vi "GUI_laptop v11c.vi"() -> ()   [LabVIEW 2019]
uses:
  <vilib>/Math Plots/3D Math Plots/3D Scatter/3D Scatter XCtrl/3D Scatter.xctl
  <vilib>/Platform/TimedLoop/XDataNode/timing_clust.ctl
  <vilib>/Platform/TimedLoop/XDataNode/nitl_modes.ctl
  <vilib>/Platform/TimedLoop/XDataNode/wakeup.ctl
  <vilib>/Analysis/_algsub.llb/Real Vector Norm.vi
  <vilib>/Instr/_visa.llb/VISA Configure Serial Port (Instr).vi
  <vilib>/Utility/file.llb/Write Delimited Spreadsheet (DBL).vi
  <vilib>/Math Plots/3D Math Plots/3D Scatter/3D Scatter Datatype/Public/Plot Helper (Vector).vi
  <vilib>/platform/TimedLoop/XDataNode/XDataNode.xnode
  <vilib>/Platform/TimedLoop/XDataNode/XDNodeRunTimeDep.lvlib
  <vilib>/Analysis/NI_AALPro.lvlib
  <vilib>/Math Plots/3D Math Plots/3D Scatter/3D Scatter Datatype/3D Scatter Datatype.lvclass
panel:
  in  "Motion Scale 4":dbl=2.0
  out "spreadsheet string":string
  out "1-D Array of Real 2":dbl[](array[numeric])
  out "1-D Array of Real":dbl[](array[numeric])
  in  "Save Path 2":path=path "C:/Users/jimmy/Documents/GitHub/Arduino-LabVIEW/zhantao/read_data_delt.csv"
  out "Numeric":i32
  out "send values":dbl[](array[numeric])
  out "Robot Feedback (xyz)":dbl[](array[numeric])
  in  "UDP Send":bool
  in  "UDP Recv":bool
  in  "L5 bound":dbl=1000.0
  in  "L4 bound (deg)":dbl=1000.0
  in  "L3 bound (mm)":dbl=1000.0
  in  "L2 bound (deg)":dbl=1000.0
  in  "L1 bound (deg)":dbl=1000.0
  in  "Joystick Type":dbl(ring) items=["Rigid Joystick", "Free Joystick"]
  out "Finished Late? [i-1]":bool
  in  "Epsilon":dbl=0.2
  out "3D Scatter":refnum<class "3D Plot Datatype.lvclass">[](xcontrol)
  out "Random Point":dbl[](array[numeric])
  out "Virtual Cursor":dbl[](array[numeric])
  out "Iteration Duration":i64
  in  "Num of Points":i32=10
  in  "z bound":dbl=2.0
  in  "y bound":dbl=5.0
  in  "x bound":dbl=5.0
  in  "Stop":bool
  in  "Round Decimals":dbl=2.0 format="%#_15g"
  in  "Save  Data":bool
  in  "Save Path":path=path "C:/Users/jimmy/Documents/GitHub/Arduino-LabVIEW/zhantao/read_data_abs.csv"
  in  "x speed":dbl=0.5
  in  "z speed":dbl=0.5
  in  "y speed":dbl=0.5
  out "error out":errorcluster
  in  "baud rate":u32=115200
  in  "VISA resource name":refnum<visa-resource-name>
  # "TODO: fix the bounds; currently bounds are arbitrary"
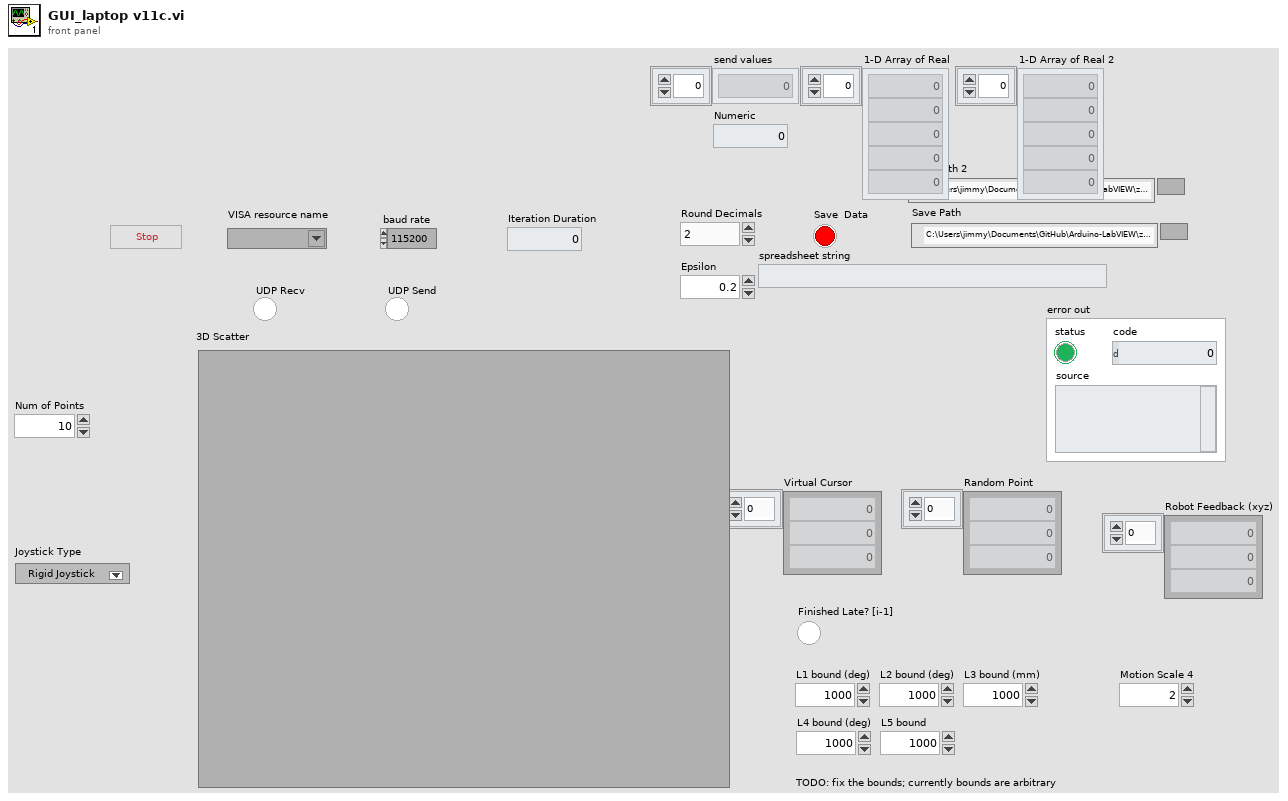
[diagram p1: front panel]
types:
  T1 = typedef "XDNodeRunTimeDep.lvlib/timing_clust.ctl" = cluster{"Expected End [f-1]":u64, "Actual End [f-1]":u64, "Finished Late? [f-1]":bool, "Expected End [i-1]":u64, "Actual End [i-1]":u64, "Finished Late? [i-1]":bool, "Expected Start [i]":u64, "Actual Start [i]":u64, "Expected Start [f]":u64, "Actual Start [f]":u64, "Source Name":string, "Structure Name":string, "Period":i64, "Deadline":i64, "Offset":i64, "Start":i64, "Priority":i32, "Timeout":i32, "Mode":T2, "Wakeup Reason":T3, "Error":errorcluster, "Source Type":string, "Secondary Source Type":string, "Global End Time":u64, "Global Start Time":u64, "Frame Duration":u64, "Iteration Duration":u64, "Assigned CPU":i32, "I/O Scan Engine Mode":u32}
  T2 = typedef "XDNodeRunTimeDep.lvlib/nitl_modes.ctl" = enum32{"No Change", "Process missed periods, maintain original phase", "Discard missed periods, maintain original phase", "Process missed periods, ignore original phase", "Discard missed periods, ignore original phase"}
  T3 = typedef "XDNodeRunTimeDep.lvlib/wakeup.ctl" = enum32{"Normal", "Aborted", "Asynchronous wakeup", "Timing source error", "Timed loop error", "Timeout"}
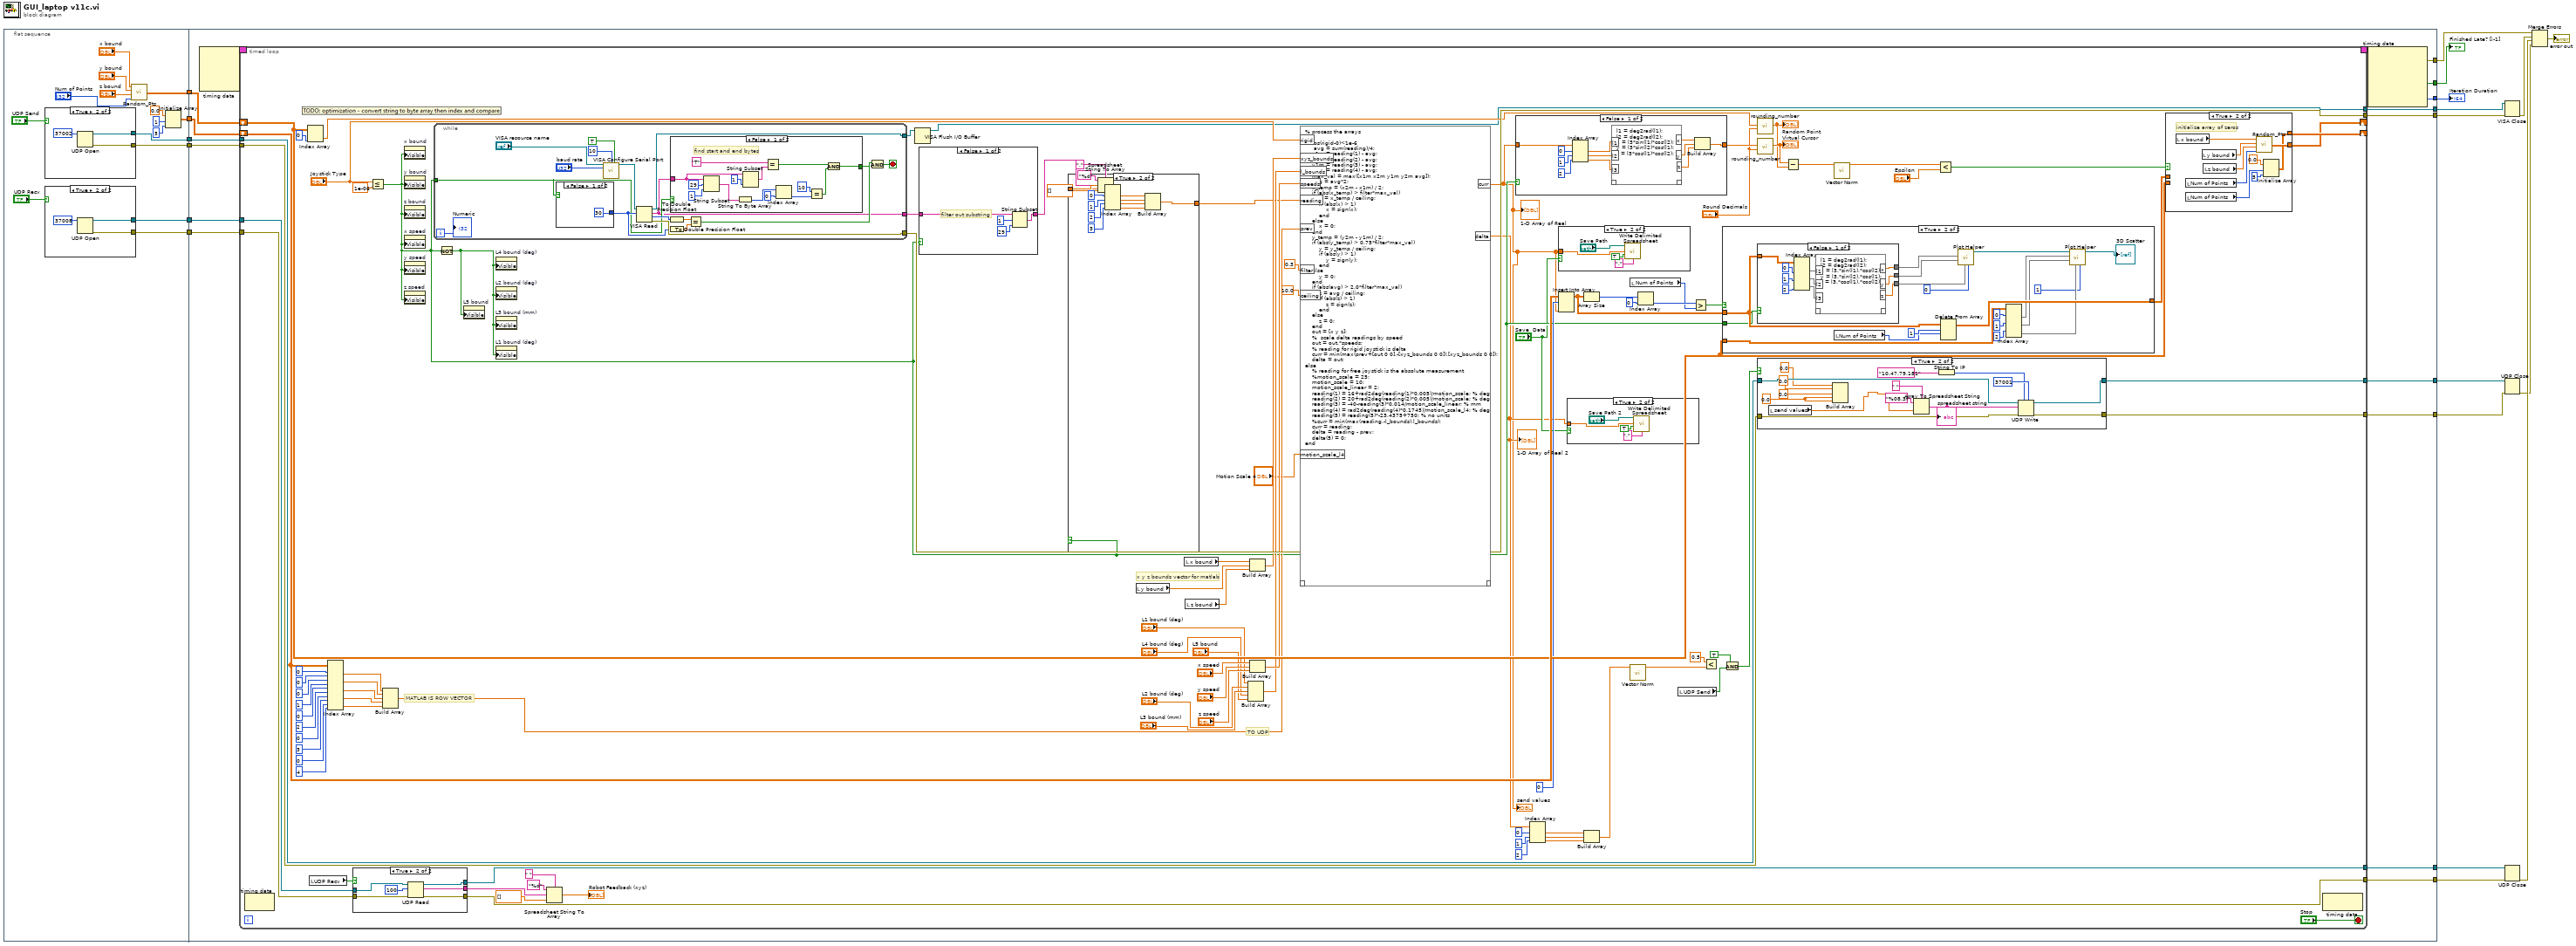
[diagram p0: block diagram]
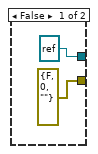
[diagram p2: hidden frame]
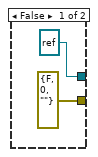
[diagram p3: hidden frame]
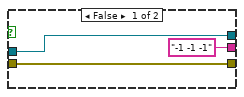
[diagram p6: hidden frame]
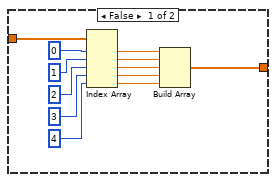
[diagram p10: hidden frame]
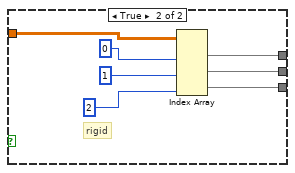
[diagram p13: hidden frame]
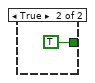
[diagram p14: hidden frame]
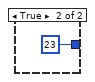
[diagram p15: hidden frame]
diagram:
  n1 = flat-sequence {
    tunnel: [w26] -> w15
    tunnel: [w30] -> w14
    tunnel: [w25] -> w13
    tunnel: [w24] -> w12
    tunnel: [w21] -> w11
    tunnel: [w20] -> w10
    tunnel: [w59] -> w19
    tunnel: [w58] -> w18
    tunnel: [w56] -> w9
    tunnel: [w54] -> w17
    tunnel: [w53] -> w16
    tunnel: w15 -> [w57]
    tunnel: w14 -> [w55]
    tunnel: w13 -> [w52]
    tunnel: w12 -> [w51]
    tunnel: w11 -> [w50]
    tunnel: w10 -> [w49]
    tunnel: [w48] -> w3
    tunnel: [w47] -> w8
    tunnel: [w46] -> w2
    tunnel: [w45] -> w1
    frame #0 {
      n2 = case shown="True" "UDP Send" {
        tunnel: [refnum<k16> refnum ("port") w38] -> w25
        tunnel: [errorcluster {"status"=FALSE, "code"=0, "source"=""} ("error out") w37] -> w20
        frame False {
        }
        frame True {
          n3 = UDP Open(11:u16 37002 ("port")) -> (port=w38:refnum<k16>, 0:w37:errorcluster)  [unwired: 4 in, 1 out]
        }
      }
      n4 = case shown="True" "UDP Recv" {
        tunnel: [refnum<k16> refnum ("port") w43] -> w24
        tunnel: [errorcluster {"status"=FALSE, "code"=0, "source"=""} ("error out") w42] -> w21
        frame False {
        }
        frame True {
          n5 = UDP Open(11:u16 37008 ("port")) -> (port=w43:refnum<k16>, 0:w42:errorcluster)  [unwired: 4 in, 1 out]
        }
      }
      n6 = call "Random_Pts.vi"("Num of Points"="Num of Points", "z bound"="z bound", "y bound"="y bound", "x bound"="x bound") -> ("appended array"=w30:dbl[][])
      n7 = Initialize Array(0.0 ("element"), 1 ("dimension size"), 5 ("dimension size")) -> (w26:dbl[][])
    }
    frame #1 {
      n8 = node-c288() -> (w61:T1)  [unwired: 4 in]
      n9 = timed-loop {
        tunnel: [w67] -> w59
        tunnel: [w159] -> w58
        shift-right: [w158] -> _
        shift-left: w57 -> [w157]
        timing: w61 -> [_]
        timing-out: [_] -> w60
        shift-right: [w153] -> _
        shift-left: w55 -> [w154]
        tunnel: w52 -> [w97]
        tunnel: w51 -> [w96]
        tunnel: w50 -> [w94]
        tunnel: w49 -> [w93]
        tunnel: [w92] -> w48
        tunnel: [w91] -> w47
        tunnel: [w90] -> w46
        tunnel: [w89] -> w45
        stop <- "Stop" stop-if-true
        # "TO UDP"
        # "MATLAB IS ROW VECTOR"
        # "x y z bounds vector for matlab"
        n10 = node-c288() -> ()  [unwired: 1 in, 1 out]
        n11 = Index Array(array=w154, index (col)=0 ("index (row)")) -> (element=w106:dbl[])  [unwired: 1 in]
        n12 = local read "UDP Recv"() -> (w95:bool)
        n13 = Index Array(array=w157, index (row) #1=0 ("disabled index (row)"), index (col) #1=0 ("disabled index (col)"), index (row) #2=0 ("disabled index (row)"), index (col) #2=1 ("disabled index (col)"), index (row) #3=0 ("disabled index (row)"), index (col) #3=2 ("disabled index (col)"), index (row) #4=0 ("disabled index (row)"), index (col) #4=3 ("disabled index (col)"), index (row) #5=0 ("disabled index (row)"), index (col) #5=4 ("disabled index (col)")) -> (element #1=w130:dbl, element #2=w129:dbl, element #3=w128:dbl, element #4=w114:dbl, element #5=w113:dbl)
        n14 = case shown="True" w95 {
          tunnel: w96 -> [w183 w190]
          tunnel: w94 -> [w184 w189]
          tunnel: [w184 w188] -> w92
          tunnel: [w183 w187] -> w90
          tunnel: ["-1 -1 -1" w185] -> w85
          frame False {
          }
          frame True {
            n15 = UDP Read(connection ID=w190, max size (548)=100, 8:w189) -> (data out=w185:string, error out=w188:errorcluster, 3:w187:refnum<k16>)  [unwired: 1 in, 2 out]
          }
        }
        n16 = Less Or Equal?(x="Joystick Type", y=1e-06) -> (x <= y?=w72:bool)
        n17 = Build Array(w130, w129, w128, w114, w113) -> (w127:dbl[])
        n18 = property on="x bound" class="DigNum (strict)"("Visible"=w72) -> ()  [unwired: 2 in, 2 out]
        n19 = property on="y bound" class="DigNum (strict)"("Visible"=w72) -> ()  [unwired: 2 in, 2 out]
        n20 = property on="z bound" class="DigNum (strict)"("Visible"=w72) -> ()  [unwired: 2 in, 2 out]
        n21 = property on="x speed" class="DigNum (strict)"("Visible"=w72) -> ()  [unwired: 2 in, 2 out]
        n22 = property on="y speed" class="DigNum (strict)"("Visible"=w72) -> ()  [unwired: 2 in, 2 out]
        n23 = property on="z speed" class="DigNum (strict)"("Visible"=w72) -> ()  [unwired: 2 in, 2 out]
        n24 = while {
          tunnel: [w283] -> w108
          tunnel: [w296] -> w159
          tunnel: [w290] -> w68
          tunnel: w72 -> [w284]
          i -> [w282]
          stop <- w286 stop-if-true
          n25 = case shown="False" w284 {
            tunnel: [30 u32 23 ("byte count")] -> w289
            frame False {
            }
            frame True {
            }
          }
          n26 = call-poly "VISA Configure Serial Port"("VISA resource name"="VISA resource name", "termination char\n(0xA = '\\n' = LF)"=u8 10 ("termination char\n(0xA = '\\n' = LF)"), "Enable Termination\nChar (T)"=TRUE ("Enable Termination\nChar (T)"), "baud rate (9600)"="baud rate") -> ("VISA resource name out"=w291:refnum<visa-resource-name>)  [unwired: 10 in, 1 out]
          n27 = VISA Read(VISA resource name=w291, byte count=w289) -> (VISA resource name out=w290:refnum<visa-resource-name>, read buffer=w283:string, return count=w298:u32, error out=w296:errorcluster)  [unwired: 1 in]
          n28 = To Double Precision Float(number=w298) -> (double precision float=w297:dbl)
          n29 = To Double Precision Float(number=w289) -> (double precision float=w288:dbl)
          n30 = case shown="False" w284 {
            tunnel: [w305 TRUE] -> w285
            tunnel: w283 -> [w308 _]
            frame False {
              # "find start and end bytes"
              n31 = String Subset(string=w308, offset (0)=29, length (rest)=1) -> (substring=w303:string)
              n32 = String To Byte Array(string=w303) -> (unsigned byte array=w302:u8[])
              n33 = String Subset(string=w308, length (rest)=1) -> (substring=w311:string)  [unwired: 1 in]
              n34 = Equal?(x="T", y=w311) -> (x = y?=w307:bool)
              n35 = Index Array(array=w302, index=0) -> (element=w300:u8)
              n36 = Equal?(x=10, y=w300) -> (x = y?=w306:bool)
              n37 = And(x=w307, y=w306) -> (x .and. y?=w305:bool)
            }
            frame True {
            }
          }
          n38 = Equal?(x=w297, y=w288) -> (x = y?=w287:bool)
          n39 = And(x=w287, y=w285) -> (x .and. y?=w286:bool)
          "Numeric" <- w282
        }
        n40 = Not(x=w72) -> (.not. x?=w71:bool)
        n41 = property on="L5 bound" class="DigNum (strict)"("Visible"=w71) -> ()  [unwired: 2 in, 2 out]
        n42 = property on="L4 bound (deg)" class="DigNum (strict)"("Visible"=w71) -> ()  [unwired: 2 in, 2 out]
        n43 = property on="L2 bound (deg)" class="DigNum (strict)"("Visible"=w71) -> ()  [unwired: 2 in, 2 out]
        n44 = property on="L3 bound (mm)" class="DigNum (strict)"("Visible"=w71) -> ()  [unwired: 2 in, 2 out]
        n45 = property on="L1 bound (deg)" class="DigNum (strict)"("Visible"=w71) -> ()  [unwired: 2 in, 2 out]
        n46 = Spreadsheet String To Array(delimiter (Tab)=" ", format string="%d", spreadsheet string=w85, array type (2D Dbl)=dbl[] []) -> (array=→"Robot Feedback (xyz)":dbl[])
        n47 = VISA Flush I/O Buffer(VISA resource name=w68) -> (VISA resource name out=w67:refnum<visa-resource-name>)  [unwired: 2 in, 1 out]
        n48 = case shown="False" w72 {
          tunnel: w108 -> [w209 w210]
          tunnel: [w206 w210] -> w107
          frame False {
            # "filter out substring"
            n49 = String Subset(string=w209, offset (0)=1, length (rest)=29) -> (substring=w206:string)
          }
          frame True {
          }
        }
        n50 = Spreadsheet String To Array(delimiter (Tab)=",", format string="%d", spreadsheet string=w107, array type (2D Dbl)=dbl[] []) -> (array=w110:dbl[])
        n51 = case shown="True" w72 {
          tunnel: w110 -> [w211 w226]
          tunnel: [w216 w225] -> w109
          frame False {
            n52 = Index Array(array=w211, index #1=0 ("Plot ID"), index #2=1 ("Plot ID"), index #3=2 ("Plot ID"), index #4=3 ("Plot ID"), index #5=4 ("Plot ID")) -> (element #1=w219:dbl, element #2=w218:dbl, element #3=w217:dbl, element #4=w213:dbl, element #5=w212:dbl)
            n53 = Build Array(w219, w218, w217, w213, w212) -> (w216:dbl[])
          }
          frame True {
            n54 = Index Array(array=w226, index #1=0 ("Plot ID"), index #2=1 ("Plot ID"), index #3=2 ("Plot ID"), index #4=3 ("index")) -> (element #1=w229:dbl, element #2=w228:dbl, element #3=w227:dbl, element #4=w223:dbl)
            n55 = Build Array(w229, w228, w227, w223) -> (w225:dbl[])
          }
        }
        n56 = local read "y bound"() -> (w132:dbl)
        n57 = local read "x bound"() -> (w133:dbl)
        n58 = local read "z bound"() -> (w131:dbl)
        n59 = Build Array("L1 bound (deg)", "L2 bound (deg)", "L3 bound (mm)", "L4 bound (deg)", "L5 bound") -> (w121:dbl[])
        n60 = Build Array(w133, w132, w131) -> (w125:dbl[])
        n61 = Build Array("x speed", "y speed", "z speed") -> (w126:dbl[])
        n62 = script code="% process the arrays\n\nif abs(rigid-0)<1e-6\n     avg = sum(reading)/4;\n    x1m = reading(1) - avg;\n    x2m = reading(2) - avg;\n    y1m = reading(3) - avg;\n    y2m = reading(4) - avg;\n    max_val = max([x1m x2m y1m y2m avg]);\n    avg = avg*2;\n    x_temp = (x2m - x1m) / 2;\n    if (abs(x_temp) > filter*max_val)\n        x = x_temp / ceiling;\n        if (abs(x) > 1)\n            x = sign(x);\n        end\n    else\n        x = 0;\n    end\n    y_temp = (y2m - y1m) / 2;\n    if (abs(y_temp) > 0.75*filter*max_val)\n        y = y_temp / ceiling;\n        if (abs(y) > 1)\n            y = sign(y);\n        end\n    else\n        y = 0;\n    end\n    if (abs(avg) > 2.0*filter*max_val)\n        z = avg / ceiling;\n        if (abs(z) > 1)\n            z = sign(z);\n        end\n    else\n        z = 0;\n    end\n    out = [x y z];\n    %  scale delta readings by speed\n    out = out.*speeds;\n    % reading for rigid joystick is delta\n    curr = min(max(prev+[out 0 0],-[xyz_bounds 0 0]),[xyz_bounds 0 0]);\n    delta = out;\nelse\n    % reading for free joystick is the absolute measurement\n    %motion_scale = 25;\n    motion_scale = 10;\n    motion_scale_linear = 2;\n    reading(1) = 16+rad2deg(reading(1)*0.005)/motion_scale; % deg\n    reading(2) = 20+rad2deg(reading(2)*0.005)/motion_scale; % deg\n    reading(3) = -40-reading(3)*0.014/motion_scale_linear; % mm\n    reading(4) = rad2deg(reading(4)*0.1745)/motion_scale_l4; % deg\n    reading(5) = reading(5)*-23.4375+750; % no units\n    %curr = min(max(reading,-l_bounds),l_bounds);\n    curr = reading;\n    delta = reading - prev;\n    delta(5) = 0;\nend"("xyz_bounds"=w125, "speeds"=w126, "reading"=w109, "prev"=w127, "rigid"="Joystick Type", "l_bounds"=w121, "filter"=0.3 ("Real"), "ceiling"=10.0 ("Real"), "motion_scale_l4"="Motion Scale 4") -> ("curr"=w63:dbl[], "delta"=w64:dbl[])  [unwired: 1 in, 1 out]
        "send values" <- w63
        "1-D Array of Real" <- w63
        "1-D Array of Real 2" <- w64
        n63 = case shown="False" w72 {
          tunnel: w63 -> [w240 w244]
          tunnel: [w233 w244] -> w155
          frame False {
            n64 = Index Array(array=w240, index #1=0 ("Plot ID"), index #2=1 ("Plot ID"), index #3=2 ("Plot ID")) -> (element #1=w239:dbl, element #2=w238:dbl, element #3=w237:dbl)
            n65 = script code="l1 = deg2rad(l1);\nl2 = deg2rad(l2);\nx = l3*sin(l1)*cos(l2);\ny = l3*sin(l2)*cos(l1);\nz = l3*cos(l1)*cos(l2);"("l1"=w239, "l2"=w238, "l3"=w237) -> ("x"=w236:dbl, "y"=w235:dbl, "z"=w234:dbl)  [unwired: 1 in, 1 out]
            n66 = Build Array(w236, w235, w234) -> (w233:dbl[])
          }
          frame True {
          }
        }
        n67 = Index Array(array=w64, index #1=0 ("disabled index (col)"), index #2=1 ("disabled index (col)"), index #3=2 ("disabled index (col)")) -> (element #1=w76:dbl, element #2=w75:dbl, element #3=w74:dbl)
        n68 = case shown="True" "Save  Data" {
          tunnel: w63 -> [_ w192]
          frame False {
          }
          frame True {
            n69 = call-poly <vilib>:"Write Delimited Spreadsheet.vi"("file path (dialog if empty)"="Save Path", "1D data"=w192, "append to file? (new file:F)"=TRUE, "delimiter (\\t)"="," ("delimiter (\\t)")) -> ()  [unwired: 10 in, 2 out]
          }
        }
        n70 = Insert Into Array(array=w157, index (row)=0, new element=w63) -> (w138:dbl[][])  [unwired: 1 in]
        n71 = case shown="True" "Save  Data" {
          tunnel: w64 -> [_ w162]
          frame False {
          }
          frame True {
            n72 = call-poly <vilib>:"Write Delimited Spreadsheet.vi"("file path (dialog if empty)"="Save Path 2", "1D data"=w162, "append to file? (new file:F)"=TRUE, "delimiter (\\t)"="," ("delimiter (\\t)")) -> ()  [unwired: 10 in, 2 out]
          }
        }
        n73 = Array Size(array=w138) -> (size(s)=w140:i32[])
        n74 = Build Array(w76, w75, w74) -> (w73:dbl[])
        n75 = local read "Num of Points"() -> (w139:i32)
        n76 = call-poly <vilib>:"Vector Norm.vi"("Input Vector"=w73) -> ("norm"=w83:dbl)  [unwired: 9 in, 1 out]
        n77 = Index Array(array=w140, index=0) -> (element=w141:i32)
        n78 = local read "UDP Send"() -> (w81:bool)
        n79 = Greater?(x=w141, y=w139) -> (0:w137:bool)
        n80 = Less?(x=0.5, y=w83) -> ()  [unwired: 1 out]
        n81 = case shown="True" w137 {
          tunnel: w138 -> [w245 w263]
          tunnel: [w245 w262] -> w156
          tunnel: w154 -> [_ w261]
          tunnel: w72 -> [_ w246]
          frame False {
          }
          frame True {
            n82 = case shown="False" w246 {
              tunnel: w263 -> [w274 w278]
              tunnel: [w265 w277] -> w252
              tunnel: [w266 w276] -> w251
              tunnel: [w267 w275] -> w250
              frame False {
                n83 = Index Array(array=w274, index (col) #1=0 ("Plot ID"), index (col) #2=1 ("Plot ID"), index (col) #3=2 ("Plot ID")) -> (element #1=w270:dbl[], element #2=w269:dbl[], element #3=w268:dbl[])  [unwired: 3 in]
                n84 = script code="l1 = deg2rad(l1);\nl2 = deg2rad(l2);\nx = l3.*sin(l1).*cos(l2);\ny = l3.*sin(l2).*cos(l1);\nz = l3.*cos(l1).*cos(l2);"("l1"=w270, "l2"=w269, "l3"=w268) -> ("x"=w265:dbl[], "y"=w266:dbl[], "z"=w267:dbl[])  [unwired: 1 in, 1 out]
              }
              frame True {
                # "rigid"
                n85 = Index Array(array=w278, index (col) #1=0 ("disabled index (col)"), index (col) #2=1 ("index (col)"), index (col) #3=2 ("index (col)")) -> (element #1=w277:dbl[], element #2=w276:dbl[], element #3=w275:dbl[])  [unwired: 3 in]
              }
            }
            n86 = local read "Num of Points"() -> (w260:i32)
            n87 = Delete From Array(array=w263, length=1, index (row)=w260) -> (array with subset deleted=w262:dbl[][])  [unwired: 1 in, 1 out]
            n88 = call-poly <vilib>:"Plot Helper.vi"("Plot ID"=0, "z vector"=w250, "y vector"=w251, "x vector"=w252) -> ("3D Plot lvclass Array out"=w254:refnum<class "3D Plot Datatype.lvclass">[])  [unwired: 2 in, 5 out]
            n89 = Index Array(array=w261, index (row) #1=0 ("index (row)"), index (row) #2=1 ("index (row)"), index (row) #3=2 ("index (row)")) -> (element #1=w258:dbl[], element #2=w257:dbl[], element #3=w256:dbl[])  [unwired: 3 in]
            n90 = call-poly <vilib>:"Plot Helper.vi"("Plot ID"=1, "z vector"=w256, "y vector"=w257, "x vector"=w258, "3D Plot lvclass Array in"=w254) -> ("3D Plot lvclass Array out"=→"3D Scatter":refnum<class "3D Plot Datatype.lvclass">[])  [unwired: 1 in, 5 out]
          }
        }
        n91 = And(x=TRUE, y=w81) -> (x .and. y?=w80:bool)
        n92 = call "rounding_number.vi"("power of ten"="Round Decimals", "Array"=w106) -> ("rounded"=w103:dbl[])  [unwired: 9 in]
        "Random Point" <- w103
        n93 = call "rounding_number.vi"("power of ten"="Round Decimals", "Array"=w155) -> ("rounded"=w104:dbl[])  [unwired: 9 in]
        "Virtual Cursor" <- w104
        n94 = case shown="True" w80 {
          tunnel: w97 -> [w165 w181]
          tunnel: w93 -> [w166 w177]
          tunnel: [w166 w173] -> w91
          tunnel: [w165 w172] -> w89
          frame False {
          }
          frame True {
            w171 = 0.0 ("element")
            n95 = local read "send values"() -> (w167:dbl[])
            n96 = Build Array(0.0 ("element"), 0.0 ("element"), 0.0 ("element"), w171, w171) -> ()  [unwired: 1 out]
            n97 = Array To Spreadsheet String(delimiter (Tab)=" ", array=w167, 3:"%08.3f" ("format string")) -> (spreadsheet string=w178:string)
            "spreadsheet string" <- w178
            n98 = String To IP(1:"10.47.79.181" ("name")) -> (0:w175:u32)
            n99 = UDP Write(address=w175, port or service name=u16 37001, connection ID=w181, data in=w178, 8:w177) -> (error out=w173:errorcluster, 3:w172:refnum<k16>)  [unwired: 1 in]
          }
        }
        n100 = Subtract(x=w104, y=w103) -> (x-y=w102:dbl[])
        n101 = call-poly <vilib>:"Vector Norm.vi"("Input Vector"=w102) -> ("norm"=w101:dbl)  [unwired: 9 in, 1 out]
        n102 = Less?(x=w101, y="Epsilon") -> (x < y?=w99:bool)
        n103 = case shown="True" w99 {
          tunnel: w154 -> [w196 _]
          tunnel: [w196 w201] -> w153
          tunnel: w156 -> [w195 _]
          tunnel: [w195 w197] -> w158
          frame False {
          }
          frame True {
            # "initialize array of zeros"
            n104 = local read "x bound"() -> (w205:dbl)
            n105 = local read "Num of Points"() -> (w202:i32)
            n106 = local read "Num of Points"() -> (w199:i32)
            n107 = local read "y bound"() -> (w204:dbl)
            n108 = local read "z bound"() -> (w203:dbl)
            n109 = call "Random_Pts.vi"("Num of Points"=w202, "z bound"=w203, "y bound"=w204, "x bound"=w205) -> ("appended array"=w201:dbl[][])
            n110 = Initialize Array(0.0 ("element"), w199, 5 ("dimension size")) -> (w197:dbl[][])
          }
        }
        n111 = node-c288() -> ()  [unwired: 1 in, 1 out]
      }
      n112 = node-c288(w60) -> (w56:errorcluster, w53:bool, w54:i64)  [unwired: 3 out]
    }
  }
  n113 = VISA Close(VISA resource name=w19, error in (no error)=w18) -> (error out=w7:errorcluster)
  n114 = UDP Close(connection ID=w1, 8:w8) -> (error out=w5:errorcluster)  [unwired: 1 out]
  n115 = UDP Close(connection ID=w2, 8:w3) -> (error out=w6:errorcluster)  [unwired: 1 out]
  n116 = Merge Errors(w9, w7, w6, w5) -> (→"error out":errorcluster)
  "Iteration Duration" <- w17
  "Finished Late? [i-1]" <- w16
